vi "TestMode_MinRecipe_20KHZ.vi"() -> ()   [LabVIEW 2017]
panel:
  out "Test Mode parameter range validation and Result":string
  out "Error output":errorcluster
  out "Test Result":picture
  out "Response Graph":cluster{dbl, u32}[](graph)
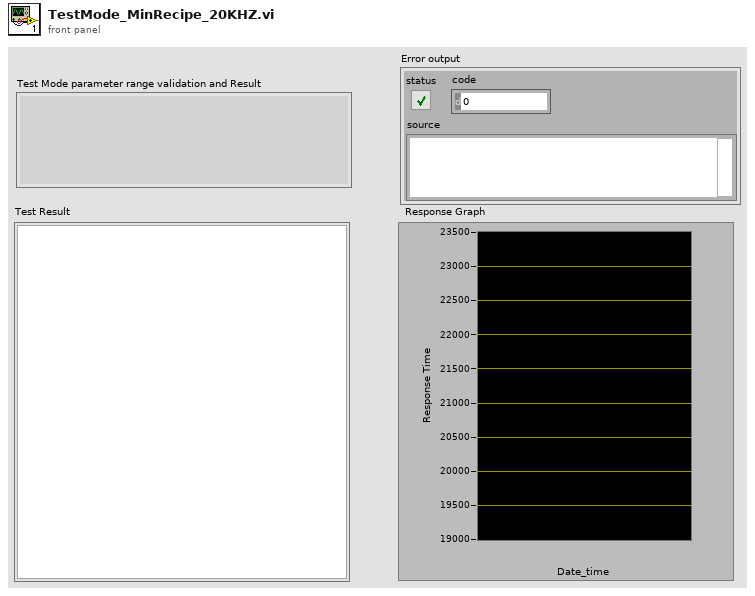
[diagram p1: front panel]
types:
  T1 = enum16{"open", "replace", "create", "open or create", "replace or create", "replace or create with confirmation"}
  T2 = cluster{"[0]":string, "[1]":string, "[2]":string, "[3]":string, "[4]":string, "[5]":string, "[6]":string, "[7]":string, "[8]":string}
  T3 = cluster{"Socket_IP_Address":string, "Socket_Port_Number":u16, "Global_ReportPath":path}
  T4 = cluster{"Iterations":u64, "DelayBetweenIterations":u32, "Timeout":u32, "MessageID":i32, "MessageLength":i32, "ResponseID":i32, "TestAmplitudeLoopC1":i32, "TestAmplitudeLoopC2":i32, "TestPhaseLoopI":i32, "TestPhaseLoopCF":i32, "TestFrequencyHigh":i32, "TestFrequencyLow":i32, "TestAmplitude":i32, "Timestamp":string, "TestSuite":string, "ReportPath":path, "FWVersionPath":path}
  T5 = typedef "imagedata.ctl" = cluster{"image type":i32, "image depth":i32, "image":u8[], "mask":u8[], "colors":u32[], "Rectangle":cluster{"left":i16, "top":i16, "right":i16, "bottom":i16}}
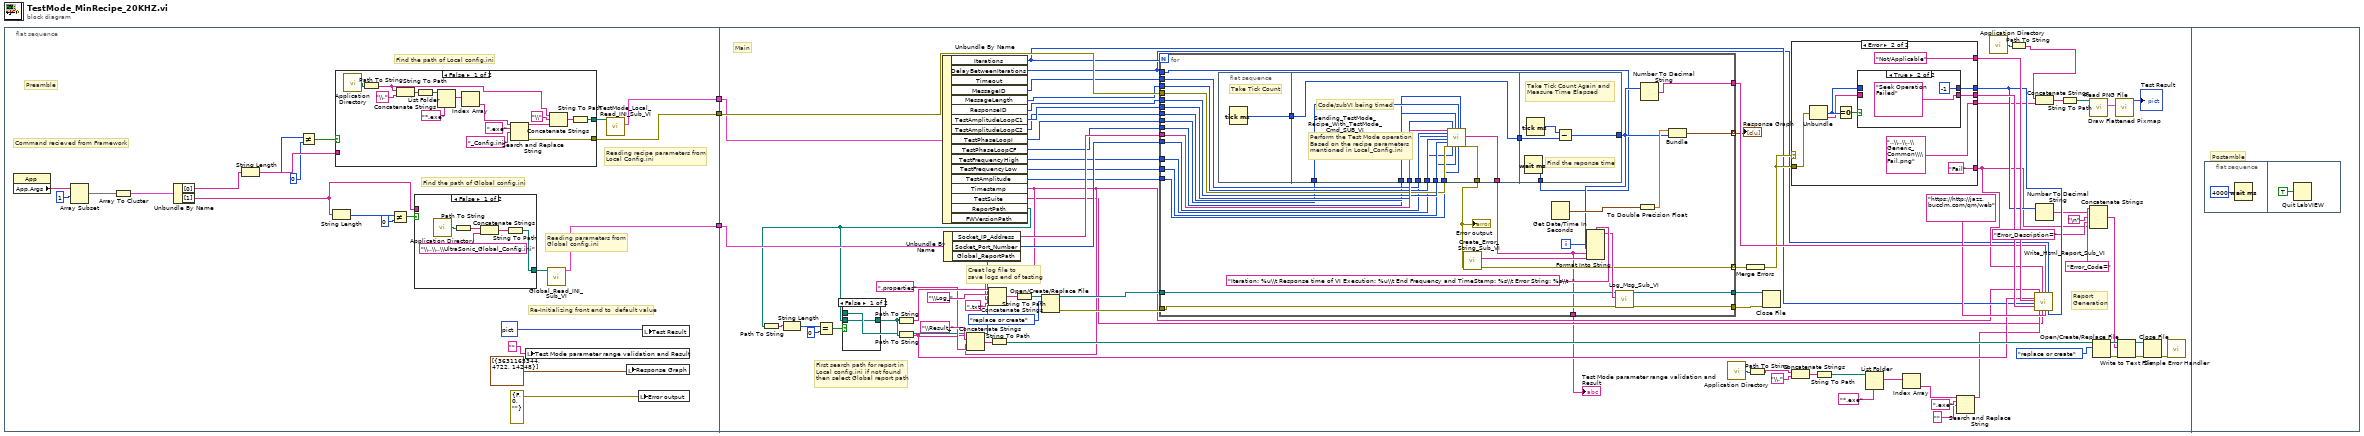
[diagram p0: block diagram]
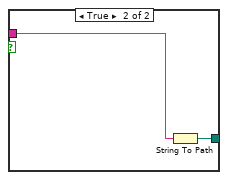
[diagram p2: hidden frame]
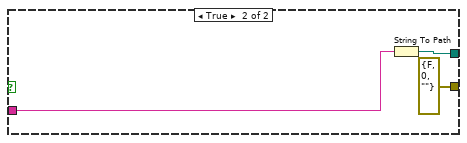
[diagram p3: hidden frame]
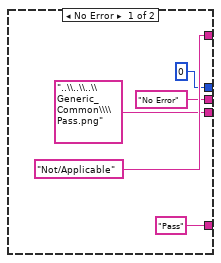
[diagram p5: hidden frame]
diagram:
  n1 = flat-sequence {
    tunnel: [w10] -> w3
    tunnel: [w9] -> w2
    tunnel: [w8] -> w1
    tunnel: w3 -> [w69]
    tunnel: w2 -> [w74]
    tunnel: w1 -> [w66]
    frame #0 {
      # "Re-Initializing front end to  default value"
      # "Reading parameters from \nGlobal config.ini"
      # "Reading recipe parameters from \nLocal Config.ini"
      # "Find the path of Global config.ini"
      # "Find the path of Local config.ini"
      # "Command recieved from Framework"
      # "Preamble"
      n2 = property class="App"() -> ("App.Args"=w12:string[])  [unwired: 2 in, 2 out]
      n3 = Array Subset "Array Subset"(array=w12, index=1) -> (w13:string[])  [unwired: 1 in]
      n4 = Array To Cluster(array=w13) -> (cluster=w14:T2)
      n5 = Unbundle By Name "Unbundle By Name"(w14) -> ("[0]"=w18:string, "[1]"=w21:string)
      n6 = String Length(string=w18) -> (length=w15:i32)
      n7 = Not Equal?(x=w15, y=0) -> (x != y?=w17:bool)
      n8 = String Length(string=w21) -> (length=w22:i32)
      n9 = case shown="False" w17 {
        tunnel: w18 -> [_ w49]
        tunnel: [w35 w48] -> w23
        tunnel: [w34 errorcluster {"status"=FALSE, "code"=0, "source"=""} ("error out")] -> w10
        frame False {
          n10 = call <vilib>:"Application Directory.vi"() -> ("Application Directory"=w33:path)
          n11 = Path To String(path=w33) -> (string=w32:string)
          n12 = Concatenate Strings(w32, "\\." ("string")) -> (w38:string)
          n13 = String To Path(string=w38) -> (path=w41:path)
          n14 = List Folder(path=w41, pattern="*.exe") -> (filenames=w37:string[])  [unwired: 2 in, 3 out]
          n15 = Index Array(array=w37) -> (element=w36:string)  [unwired: 1 in]
          n16 = Search and Replace String(input string=w36, search string=".exe", replace string="_Config.ini" ("replace string (\"\")")) -> (result string=w44:string, error out=w34:errorcluster)  [unwired: 5 in, 2 out]
          n17 = Concatenate Strings(w32, "\\" ("string"), w44) -> (w42:string)
          n18 = String To Path(string=w42) -> (path=w35:path)
        }
        frame True {
          n19 = String To Path(string=w49) -> (path=w48:path)
        }
      }
      n20 = Not Equal?(x=w22, y=0) -> (x != y?=w20:bool)
      n21 = case shown="False" w20 {
        tunnel: [w27 w31] -> w24
        tunnel: w21 -> [_ w30]
        frame False {
          n22 = call <vilib>:"Application Directory.vi"() -> ("Application Directory"=w26:path)
          n23 = Path To String(path=w26) -> (string=w25:string)
          n24 = Concatenate Strings(w25, "\\..\\..\\UltraSonic_Global_Config.ini" ("string")) -> (w28:string)
          n25 = String To Path(string=w28) -> (path=w27:path)
        }
        frame True {
          n26 = String To Path(string=w30) -> (path=w31:path)
        }
      }
      n27 = local write "Test Mode parameter range validation and Result"("" ("Test Mode parameter range validation and Result")) -> ()
      n28 = call "Global_Read_INI_Sub_VI.vi"("Config File Path"=w24) -> ("output cluster"=w9:T3)  [unwired: 14 in]
      n29 = call "TestMode_Local_Read_INI_Sub_VI.vi"("Config File Path"=w23) -> ("output cluster"=w8:T4)  [unwired: 10 in]
      n30 = local write "Response Graph"(cluster{dbl, u32}[] [{3631165344.4722, 14248}] ("Response Graph")) -> ()
      n31 = local write "Error output"(errorcluster {"status"=FALSE, "code"=0, "source"=""} ("Error output")) -> ()
      n32 = local write "Test Result"(picture data[5B] ("Test Result")) -> ()
    }
    frame #1 {
      # "Report \nGeneration"
      # "Creat log file to \nsave logs end of testing"
      # "First search path for report in\nLocal config.ini if not found\nthen select Global report path"
      # "Main"
      n33 = Unbundle By Name(w66) -> ("Iterations"=w68:u64, "DelayBetweenIterations"=w67:u32, "MessageID"=w65:i32, "MessageLength"=w64:i32, "ResponseID"=w63:i32, "TestAmplitudeLoopC1"=w62:i32, "TestAmplitudeLoopC2"=w61:i32, "TestPhaseLoopI"=w60:i32, "TestPhaseLoopCF"=w59:i32, "TestFrequencyHigh"=w58:i32, "TestFrequencyLow"=w57:i32, "TestAmplitude"=w56:i32, "Timestamp"=w55:string, "TestSuite"=w54:string, "ReportPath"=w53:path)  [unwired: 2 out]
      n34 = Path To String(path=w53) -> (string=w119:string)
      n35 = String Length(string=w119) -> (length=w118:i32)
      n36 = Equal?(x=w118, y=0) -> (x = y?=w116:bool)
      n37 = Unbundle By Name(w74) -> ("Socket_IP_Address"=w72:string, "Socket_Port_Number"=w71:u16, "Global_ReportPath"=w73:path)
      n38 = case shown="False" w116 {
        tunnel: w73 -> [_ w131]
        tunnel: [w130 w131] -> w115
        tunnel: w53 -> [w130 _]
        frame False {
        }
        frame True {
        }
      }
      n39 = Path To String(path=w115) -> (string=w121:string)
      n40 = Path To String(path=w115) -> (string=w92:string)
      n41 = Concatenate Strings(w92, "\\Result_" ("string"), w55, ".properties" ("string")) -> (w113:string)
      n42 = Concatenate Strings(w121, "\\Log_" ("string"), w55, ".txt" ("string")) -> (w124:string)
      n43 = String To Path(string=w113) -> (path=w105:path)
      n44 = String To Path(string=w124) -> (path=w123:path)
      n45 = Open/Create/Replace File(file path (use dialog)=w123, operation (0:open)=T1."replace or create") -> (refnum out=w93:refnum<file>, error out=w96:errorcluster)  [unwired: 1 in, 4 out]
      n46 = for {
        N: w68 -> [_]
        tunnel: [w161] -> w127
        tunnel: w93 -> [w155]
        tunnel: [w154] -> w95
        tunnel: [w152] -> w94
        tunnel: [w157] -> w125 mode=indexing
        tunnel: w96 -> [w153]
        tunnel: [w149] -> w91 mode=indexing
        tunnel: w72 -> [w148]
        tunnel: w71 -> [w141]
        tunnel: w65 -> [w147]
        tunnel: w64 -> [w146]
        tunnel: w63 -> [w145]
        tunnel: w67 -> [w144]
        tunnel: w69 -> [w142]
        tunnel: w62 -> [w140]
        tunnel: w61 -> [w139]
        tunnel: w60 -> [w138]
        tunnel: w59 -> [w137]
        tunnel: w58 -> [w136]
        tunnel: w57 -> [w135]
        tunnel: w56 -> [w134]
        tunnel: [w132] -> w52
        i -> [w150]
        n47 = flat-sequence {
          tunnel: [w164] -> w163
          tunnel: [w180] -> w162
          tunnel: w163 -> [w180]
          tunnel: w148 -> [w179]
          tunnel: w141 -> [w178]
          tunnel: w147 -> [w177]
          tunnel: w146 -> [w176]
          tunnel: w145 -> [w175]
          tunnel: w142 -> [w174]
          tunnel: w140 -> [w173]
          tunnel: w139 -> [w172]
          tunnel: w138 -> [w171]
          tunnel: w137 -> [w170]
          tunnel: w136 -> [w169]
          tunnel: w135 -> [w168]
          tunnel: w134 -> [w167]
          tunnel: [w165] -> w132
          tunnel: [w166] -> w133
          tunnel: w162 -> [w184]
          tunnel: [w182] -> w151
          tunnel: w144 -> [w181]
          frame #0 {
            # "Take Tick Count"
            n48 = Tick Count (ms)() -> (millisecond timer value=w164:u32)
          }
          frame #1 {
            # "Perform the Test Mode operation\nBased on the recipe parameters\nmentioned in Local_Config.ini"
            # "Code/subVI being timed"
            n49 = call "Sending_TestMode_Recipe_With_TestMode_Cmd_SUB_VI.vi"("Socket IP Address"=w179, "Socket Port Number"=w178, "Receipe Msg ID"=w177, "Receipe Message length"=w176, "Response ID"=w175, "error in (no error)"=w174, "TestAmplitudeLoopC1"=w173, "TestFrequencyHigh"=w169, "TestAmplitudeLoopC2"=w172, "TestFrequencyLow"=w168, "TestPhaseLoopI"=w171, "TestAmplitude"=w167, "TestPhaseLoopCF"=w170) -> ("Test Mode Signature"=w165:string, "error out"=w166:errorcluster)  [unwired: 5 in]
          }
          frame #2 {
            # "Find the reponse time"
            # "Take Tick Count Again and Measure Time Elapsed"
            n50 = Wait (ms)(milliseconds to wait=w181) -> ()  [unwired: 1 out]
            n51 = Tick Count (ms)() -> (millisecond timer value=w183:u32)
            n52 = Subtract(x=w183, y=w184) -> (x-y=w182:u32)
          }
        }
        n53 = call "Create_Error_String_Sub_VI.vi"("error in"=w133) -> ("error out"=w149:errorcluster, "Error String"=w143:string)  [unwired: 9 in]
        n54 = Get Date/Time In Seconds() -> (seconds since 1Jan1904=w158:timestamp)
        n55 = Format Into String(format string="Iteration: %u\\t Response time of VI Execution: %u\\t End Frequency and TimeStamp: %s\\t Error String: %s\\t  ", w150, w151, w132, w143) -> (resulting string=w156:string)  [unwired: 2 in, 1 out]
        n56 = call "Log_Msg_Sub_VI.vi"("error in (no error)"=w153, "String"=w156, "Byte Stream File in"=w155) -> ("error out"=w152:errorcluster, "Byte Stream File out"=w154:refnum<file>)  [unwired: 7 in]
        n57 = To Double Precision Float(number=w158) -> (double precision float=w159:dbl)
        n58 = Number To Decimal String(number=w151) -> (decimal integer string=w161:string)  [unwired: 1 in]
        n59 = Bundle "Bundle"(w159, w151) -> (w157:cluster{dbl, u32})  [unwired: 1 in]
        "Error output" <- w133
      }
      "Response Graph" <- w125
      "Test Mode parameter range validation and Result" <- w52
      n60 = call <vilib>:"Application Directory.vi"() -> ("Application Directory"=w88:path)
      n61 = Merge Errors "Merge Errors"(w91) -> (w70:errorcluster)
      n62 = Path To String(path=w88) -> (string=w51:string)
      n63 = Close File(refnum=w95, error in=w94) -> ()  [unwired: 2 out]
      n64 = Concatenate Strings(w51, "\\." ("string")) -> (w86:string)
      n65 = case shown="Error" w70 {
        tunnel: ["Pass" "Fail"] -> w97
        tunnel: w70 -> [_ w196]
        tunnel: [0 ("code") w192] -> w101
        tunnel: ["No Error" ("source") w193] -> w129
        tunnel: ["Not/Applicable" "Not/Applicable"] -> w128
        tunnel: ["..\\..\\..\\Generic_Common\\\\Pass.png" ("string") "..\\..\\..\\Generic_Common\\\\Fail.png" ("string")] -> w75
        frame No Error {
        }
        frame Error {
          n66 = Unbundle(w196) -> ("code"=w194:i32, "source"=w190:string)  [unwired: 1 out]
          n67 = Equal To 0?(x=w194) -> (x = 0?=w191:bool)
          n68 = case shown="True" w191 {
            tunnel: [w200 -1 ("code")] -> w192
            tunnel: [w199 "Seek Operation Failed" ("source")] -> w193
            tunnel: w194 -> [w200 _]
            tunnel: w190 -> [w199 _]
            frame False {
            }
            frame True {
            }
          }
        }
      }
      n69 = String To Path(string=w86) -> (path=w90:path)
      n70 = List Folder(path=w90, pattern="*.exe") -> (filenames=w85:string[])  [unwired: 2 in, 3 out]
      n71 = Index Array(array=w85) -> (element=w81:string)  [unwired: 1 in]
      n72 = Search and Replace String(input string=w81, search string=".exe", replace string="" ("replace string (\"\")")) -> (result string=w84:string)  [unwired: 5 in, 3 out]
      n73 = call <vilib>:"Application Directory.vi"() -> ("Application Directory"=w76:path)
      n74 = Path To String(path=w76) -> (string=w50:string)
      n75 = call "Write_Html_Report_Sub_VI.vi"("ReprtPath"=w92, "Remarks"=w128, "Iterations"=w68, "Error Description"=w129, "Timestamp"=w55, "TestCase"=w84, "Verdict"=w97, "TestSuite"=w54, "Time taken to execute  test in msec"=w127, "JazzDashboardLink"="https://http://jazz.bucclm.com/qm/web" ("TestSuite"), "Delay Between Iterations"=w67, "Error Code"=w101) -> ()  [unwired: 8 in]
      n76 = Concatenate Strings(w50, w75) -> (w77:string)
      n77 = Number To Decimal String(number=w101) -> (decimal integer string=w100:string)  [unwired: 1 in]
      n78 = String To Path(string=w77) -> (path=w80:path)
      n79 = call <vilib>:"Read PNG File.vi"("path to PNG file"=w80) -> ("image data"=w78:T5)  [unwired: 8 in, 2 out]
      n80 = Concatenate Strings("Error_Code=" ("string"), w100, "\n", "Error_Description=" ("string"), w97) -> (w103:string)
      n81 = Open/Create/Replace File(file path (use dialog)=w105, operation (0:open)=T1."replace or create") -> (refnum out=w104:refnum<file>, error out=w109:errorcluster)  [unwired: 4 in, 1 out]
      n82 = call <vilib>:"Draw Flattened Pixmap.vi"("image data"=w78) -> ("new picture"=→"Test Result":picture)  [unwired: 8 in]
      n83 = Write to Text File(file (use dialog)=w104, text=w103, error in=w109) -> (refnum out=w108:refnum<file>, error out=w107:errorcluster)  [unwired: 1 in, 1 out]
      n84 = Close File(refnum=w108, error in=w107) -> (error out=w106:errorcluster)  [unwired: 1 out]
      n85 = call <vilib>:"Simple Error Handler.vi"("error in (no error)"=w106) -> ()  [unwired: 4 in, 5 out]
    }
    frame #2 {
      # "Postamble"
      n86 = flat-sequence {
        frame #0 {
          n87 = Wait (ms)(milliseconds to wait=u32 4000) -> ()  [unwired: 1 out]
        }
        frame #1 {
          n88 = Quit LabVIEW(quit? (T)=TRUE) -> ()
        }
      }
    }
  }
